vi "ToString_ReturnsVITitleAndDataName.vi"() -> ()   [LabVIEW 2017, in "Theory.Tests.lvlib"]
uses:
  Theory.Tests.lvlib
  ControlData.ctl
  2f3da0ef-3c9e-445a-9256-49f9cfd4a406.vi
  Constraint/IsEqual/Create.vi
  Theory/Theory.lvclass
  Constraint/IsEqual/IsEqual.lvclass
  Support/Support.lvlib
panel:
  out "error out":errorcluster
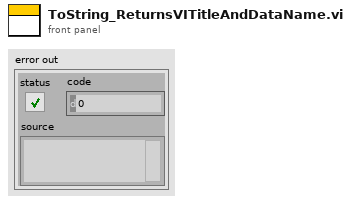
[diagram p1: front panel]
types:
  T1 = typedef "ControlData.ctl" = cluster{"Name":string, "Data":variant}
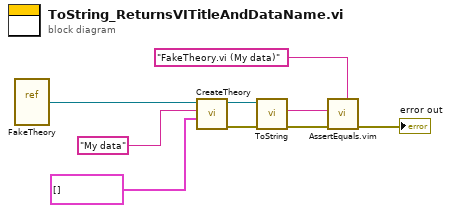
[diagram p0: block diagram]
diagram:
  n1 = vi-ref "FakeTheory.vi"() -> (w4:refnum<vi>)
  n2 = call "CreateTheory.vi"("Control Data"=T1[] [] ("Array"), "Data Name (\"\")"="My data" ("Data Name (\"\")"), "VI Refnum"=w4) -> ("error out"=w8:errorcluster, "Theory"=w9:refnum<class "Theory.lvclass">)  [unwired: 7 in]
  n3 = call-dynamic "ToString.vi"("error in (no error)"=w8, "Theory in"=w9) -> ("error out"=w7:errorcluster, "String"=w3:string)  [unwired: 7 in, 1 out]
  n4 = call "AssertEquals.vim"("Expected"="FakeTheory.vi (My data)" ("Data Name (\"\")"), "error in (no error)"=w7, "Actual"=w3) -> ("error out"=→"error out":errorcluster)  [unwired: 8 in]
